vi "ShiftRegister.vi"() -> ()   [LabVIEW 2015]
panel:
  out "Numeric 4":i32
  out "Numeric 3":i32
  out "Array 2":i32[](array[numeric])
  out "Numeric 2":i32
  out "Numeric":i32
  out "Array":i32[](array[numeric])
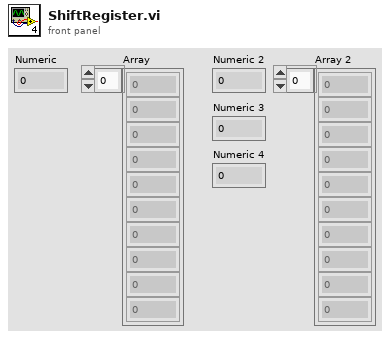
[diagram p1: front panel]
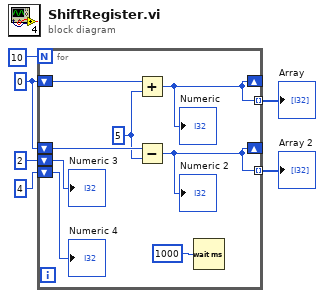
[diagram p0: block diagram]
diagram:
  w3 = 0
  n1 = for {
    N: 10 -> [_]
    shift-right: [w13] -> _
    shift-left: w3 -> [w14]
    tunnel: [w13] -> w5 mode=indexing
    shift-right: [w9] -> _
    shift-left: w3 -> [w11]
    tunnel: [w9] -> w4 mode=indexing
    shift-left: 2 -> [w8]
    shift-left: 4 -> [w7]
    w10 = 5 ("y")
    n2 = Add(x=w14, y=w10) -> (x+y=w13:i32)
    "Numeric" <- w13
    n3 = Subtract(x=w11, y=w10) -> (x-y=w9:i32)
    "Numeric 2" <- w9
    n4 = Wait (ms)(milliseconds to wait=u32 1000) -> ()  [unwired: 1 out]
    "Numeric 3" <- w8
    "Numeric 4" <- w7
  }
  "Array" <- w5
  "Array 2" <- w4
